vi "Test Mixer.vi"(8 "error in (no error)":errorcluster, 11 "DSP.lvclass":refnum<class "DSP.lvclass">) -> (0 "error out":errorcluster, 3 "DSP.lvclass":refnum<class "DSP.lvclass">)   [LabVIEW 2019, in "DSP.lvclass"]
uses:
  DSP.lvclass
  Typedefs/REF.Channel--Cluster--Array.ctl
  Typedefs/REF.Channel--Cluster.ctl
  Typedefs/AI.Channel--Cluster--Array.ctl
  Typedefs/AI.Channel--Cluster.ctl
  Typedefs/DSP.Config.Timing--Cluster.ctl
  DSP.lvclass/DSP.ctl
  <vilib>/measure/NI_MABase.lvlib
panel:
  in  "AI Channels":T1=[{"Enable?"=TRUE, "Channel"=1, "References"=[1], "reference index"=0}] {"reference index" min=1; "References" items=["", "1", "2", "3"]; "Channel" min=1}
  out "Waveform Chart":dbl[](graph)
  out "key":string="AI1.Ref1.X"
  in  "index":i32=2
  out "phase out":dbl[](array[numeric])=[324.00000000000387, 61.19999999999811]
  out "Waveform 2":waveform(dbl)[](graph)
  in  "frequency":dbl[](array[numeric])=[13.0, 9.9] format="%0.2p"
  in  "REF Channels 2":T3=[{"Enable?"=TRUE, "Channel"=1, "Frequency"=13.0, "Phase"=0.0, "TC"=0.3, "Roll-Off"=2}] {"Roll-Off" min=1; "TC" min=0.0001 format="%#_3p"; "Phase" format="%.3g"; "Frequency" min=0.0001 max=10000.0 format="%.3g"; "Channel" min=1}
  out "Waveform 1":waveform(dbl)[](graph)
  in  "stop":bool
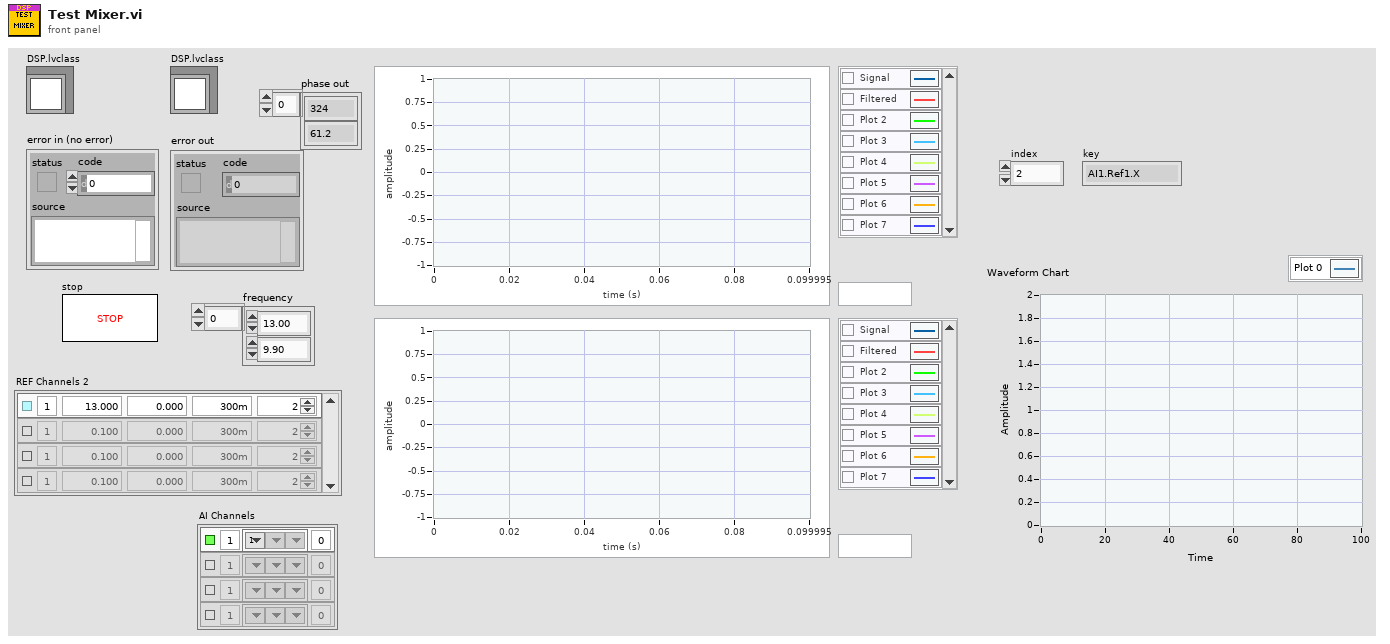
[diagram p1: front panel]
types:
  T1 = typedef "DSP.lvclass/AI.Channel--Cluster--Array.ctl" = T2[]
  T2 = typedef "DSP.lvclass/AI.Channel--Cluster.ctl" = cluster{"Enable?":bool, "Channel":i32, "References":i32[], "reference index":i32}
  T3 = typedef "DSP.lvclass/REF.Channel--Cluster--Array.ctl" = T4[]
  T4 = typedef "DSP.lvclass/REF.Channel--Cluster.ctl" = cluster{"Enable?":bool, "Channel":i32, "Frequency":dbl, "Phase":dbl, "TC":dbl, "Roll-Off":i32}
  T5 = typedef "DSP.lvclass/DSP.Config.Timing--Cluster.ctl" = cluster{"Sampling":cluster{"Fs":dbl, "#s":i32}, "Fs_Out":dbl}
  T6 = cluster{"AO":waveform(dbl)[], "AI":waveform(dbl)[], "Ref_X":waveform(dbl)[], "Ref_Y":waveform(dbl)[], "X":waveform(dbl)[], "Y":waveform(dbl)[]}
  T7 = typedef "DSP.lvclass/Results--Cluster.ctl" = cluster{"Time Stamp":timestamp, "Results (Dictionary)":T8[]}
  T8 = typedef "DSP.lvclass/Results Dictionary--Cluster.ctl" = cluster{"key":string, "value":dbl[]}
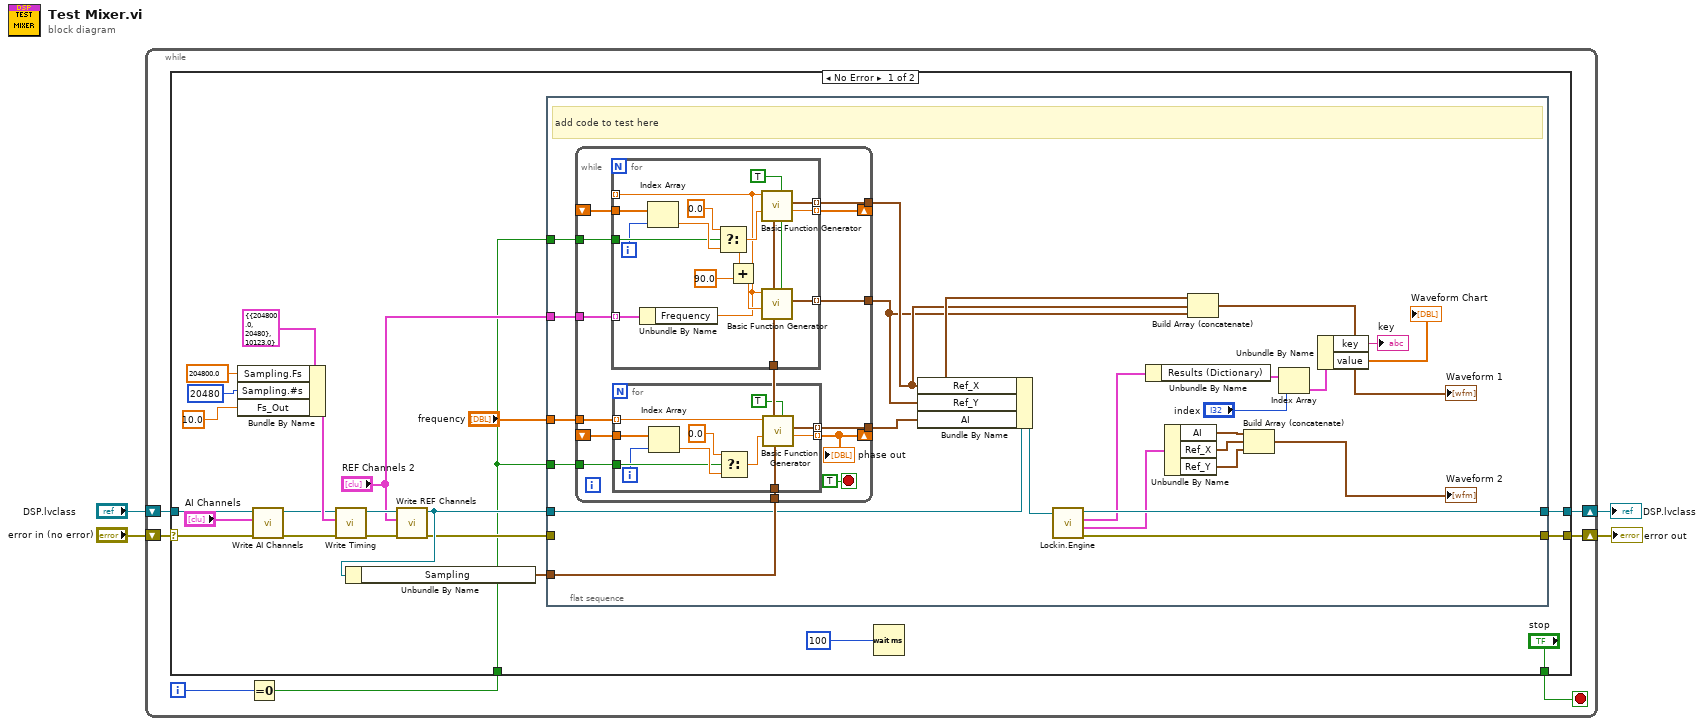
[diagram p0: block diagram]
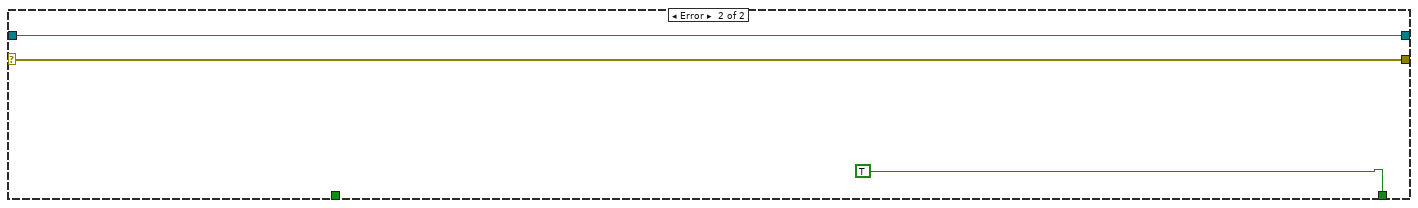
[diagram p2: hidden frame]
diagram:
  n1 = while {
    shift-right: [w10] -> w3
    shift-left: "error in (no error)" -> [w11]
    shift-right: [w8] -> w1
    shift-left: "DSP.lvclass" -> [w9]
    i -> [w7]
    stop <- w6 stop-if-true
    n2 = Equal To 0?(x=w7) -> (x = 0?=w5:bool)
    n3 = case shown="No Error" w11 {
      selector: w11 -> [w16 w99]
      tunnel: [w32 w99] -> w10
      tunnel: [w33 w98] -> w8
      tunnel: w9 -> [w14 w98]
      tunnel: ["stop" TRUE ("stop")] -> w6
      tunnel: w5 -> [w18 _]
      frame No Error {
        n4 = Bundle By Name(cluster=T5 {"Sampling"={"Fs"=204800.0, "#s"=20480}, "Fs_Out"=10123.0} ("Timing"), "Sampling.Fs"=204800.0, "Sampling.#s"=20480, "Fs_Out"=10.0) -> (w20:T5)
        n5 = call "Write AI Channels.vi"("error in (no error)"=w16, "AI Channels"="AI Channels", "DSP in"=w14) -> ("error out"=w15:errorcluster, "DSP out"=w17:refnum<class "DSP.lvclass">)  [unwired: 7 in]
        n6 = call "Write Timing.vi"("error in (no error)"=w15, "Timing"=w20, "DSP in"=w17) -> ("error out"=w26:errorcluster, "DSP out"=w27:refnum<class "DSP.lvclass">)  [unwired: 7 in]
        n7 = call "Write REF Channels.vi"("error in (no error)"=w26, "REF Channels"="REF Channels 2", "DSP in"=w27) -> ("error out"=w29:errorcluster, "DSP out"=w30:refnum<class "DSP.lvclass">)  [unwired: 7 in]
        n8 = Unbundle By Name(w30) -> ("Sampling"=w25:cluster{"Fs":dbl, "#s":i32})
        n9 = flat-sequence {
          tunnel: [w54] -> w33
          tunnel: w29 -> [_]
          tunnel: [w53] -> w32
          tunnel: w30 -> [w52]
          tunnel: "frequency" -> [w57]
          tunnel: w25 -> [w56]
          tunnel: w18 -> [w55]
          tunnel: "REF Channels 2" -> [w50]
          tunnel: w18 -> [w49]
          frame #0 {
            # "add code to test here"
            n10 = while {
              tunnel: w57 -> [w70]
              tunnel: w56 -> [w64]
              tunnel: [w69] -> w43
              shift-right: [w68] -> _
              shift-left: _ -> [w67]
              tunnel: w55 -> [w65]
              tunnel: [w63] -> w42
              tunnel: [w62] -> w41
              shift-right: [w61] -> _
              shift-left: _ -> [w60]
              tunnel: w50 -> [w59]
              tunnel: w49 -> [w58]
              stop <- TRUE stop-if-true
              n11 = for {
                tunnel: [w85] -> w63 mode=indexing
                tunnel: [w71] -> _ mode=indexing
                tunnel: w64 -> [w77]
                tunnel: [w84] -> w61 mode=indexing
                tunnel: w60 -> [w83]
                tunnel: w58 -> [w80]
                tunnel: [w76] -> w62 mode=indexing
                tunnel: w59 -> [w75] mode=indexing
                i -> [w79]
                w78 = TRUE ("reset signal")
                n12 = Unbundle By Name(w75) -> ("Frequency"=w71:dbl)
                n13 = Index Array(array=w83, index=w79) -> (element=w81:dbl)
                n14 = Select(t=0.0, s=w80, f=w81) -> (s? t:f=w74:dbl)
                n15 = Add(x=w74, y=90.0) -> (x+y=w72:dbl)
                n16 = call <vilib>:"Basic Function Generator.vi"("reset signal"=w78, "sampling info"=w77, "phase"=w74, "frequency"=w71) -> ("phase out"=w84:dbl, "signal out"=w85:waveform(dbl))  [unwired: 5 in, 1 out]
                n17 = call <vilib>:"Basic Function Generator.vi"("reset signal"=w78, "sampling info"=w77, "phase"=w72, "frequency"=w71) -> ("signal out"=w76:waveform(dbl))  [unwired: 5 in, 2 out]
              }
              n18 = for {
                tunnel: [w96] -> w69 mode=indexing
                tunnel: w70 -> [w95] mode=indexing
                tunnel: w64 -> [w94]
                tunnel: [w93] -> w68 mode=indexing
                tunnel: w67 -> [w92]
                tunnel: w65 -> [w87]
                i -> [w86]
                n19 = Index Array(array=w92, index=w86) -> (element=w89:dbl)
                n20 = Select(t=0.0, s=w87, f=w89) -> (s? t:f=w90:dbl)
                n21 = call <vilib>:"Basic Function Generator.vi"("reset signal"=TRUE, "sampling info"=w94, "phase"=w90, "frequency"=w95) -> ("phase out"=w93:dbl, "signal out"=w96:waveform(dbl))  [unwired: 5 in, 1 out]
              }
              "phase out" <- w68
            }
            n22 = Bundle By Name(cluster=w52, "Ref_X"=w42, "Ref_Y"=w41, "AI"=w43) -> (w51:refnum<class "DSP.lvclass">)
            n23 = call "Lockin.Engine.vi"("DSP in"=w51) -> ("error out"=w53:errorcluster, "Downsampled Waveforms"=w48:T6, "Results"=w39:T7, "DSP out"=w54:refnum<class "DSP.lvclass">)  [unwired: 6 in, 1 out]
            n24 = Unbundle By Name(w39) -> ("Results (Dictionary)"=w38:T8[])
            n25 = Unbundle By Name(w48) -> ("AI"=w45:waveform(dbl)[], "Ref_X"=w47:waveform(dbl)[], "Ref_Y"=w46:waveform(dbl)[])
            n26 = Build Array (concatenate)(w43, w42, w41) -> (→"Waveform 1":waveform(dbl)[])
            n27 = Build Array (concatenate)(w45, w47, w46) -> (→"Waveform 2":waveform(dbl)[])
            n28 = Index Array(array=w38, index="index") -> (element=w36:T8)
            n29 = Unbundle By Name(w36) -> ("key"=→"key":string, "value"=→"Waveform Chart":dbl[])
          }
        }
        n30 = Wait (ms)(milliseconds to wait=u32 100) -> ()  [unwired: 1 out]
      }
      frame Error {
      }
    }
  }
  "error out" <- w3
  "DSP.lvclass" <- w1
